vi "LVUSBRH2_VISA_SendCommand.vi"(8 "error in (no error)":errorcluster caption="error in(no errro)", 10 "cmd string":string="getrh", 11 "VISA rssc":refnum<visa-resource-name>) -> (0 "error out":errorcluster, 3 "VISA rssc out":refnum<visa-resource-name>)   [LabVIEW 2020]
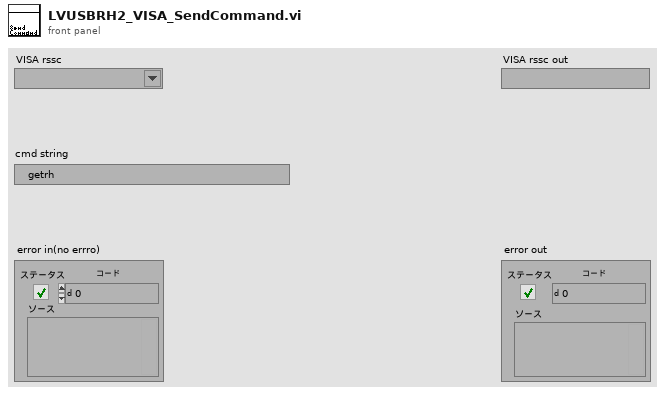
[diagram p1: front panel]
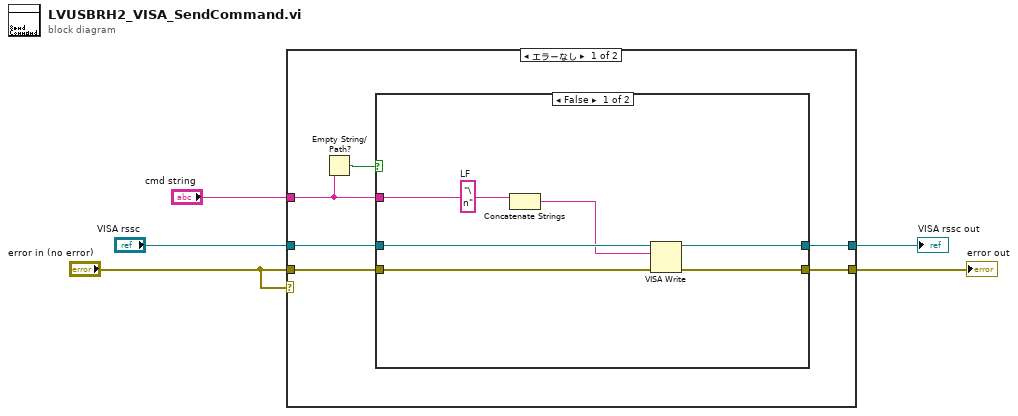
[diagram p0: block diagram]
diagram:
  n1 = case shown="エラーなし" "error in (no error)" {
    tunnel: "VISA rssc" -> [w11 w22]
    tunnel: [w10 w22] -> w4
    tunnel: "error in (no error)" -> [w9 w21]
    tunnel: [w8 w21] -> w3
    tunnel: "cmd string" -> [w7 _]
    frame No Error {
      n2 = Empty String/Path?(string/path=w7) -> (empty?=w6:bool)
      n3 = case shown="FALSE" w6 {
        tunnel: w11 -> [w18 w20]
        tunnel: [w17 w20] -> w10
        tunnel: w9 -> [w16 w19]
        tunnel: [w15 w19] -> w8
        tunnel: w7 -> [w13 _]
        frame False {
          w12 = "\n"  # LF
          n4 = Concatenate Strings(w13, w12) -> (w14:string)
          n5 = VISA Write(VISA resource name=w18, write buffer=w14, error in (no error)=w16) -> (VISA resource name out=w17:refnum<visa-resource-name>, error out=w15:errorcluster)  [unwired: 1 out]
        }
        frame True {
        }
      }
    }
    frame Error {
    }
  }
  "VISA rssc out" <- w4
  "error out" <- w3
